vi "Buffer ArrayShellTest.vi"() -> ()   [LabVIEW 2014]
uses:
  <vilib>/measure/mamon.llb/Trigger Detection for 1 Channel.vi
  <vilib>/measure/NI_MAPro.lvlib
panel:
  out "Array":dbl[](array[numeric])
  out "trigger location":dbl
  out "index of element":i32
  out "Output Graph":dynamicdata(graph) caption="Sine"
  in  "stop":bool
  out "Output Array":dbl[](array[numeric])
  in  "Total amount of Pts":i32
  in  "Trigger Threshold":dbl
  out "SineGenerator":dynamicdata(graph) caption="Sine"
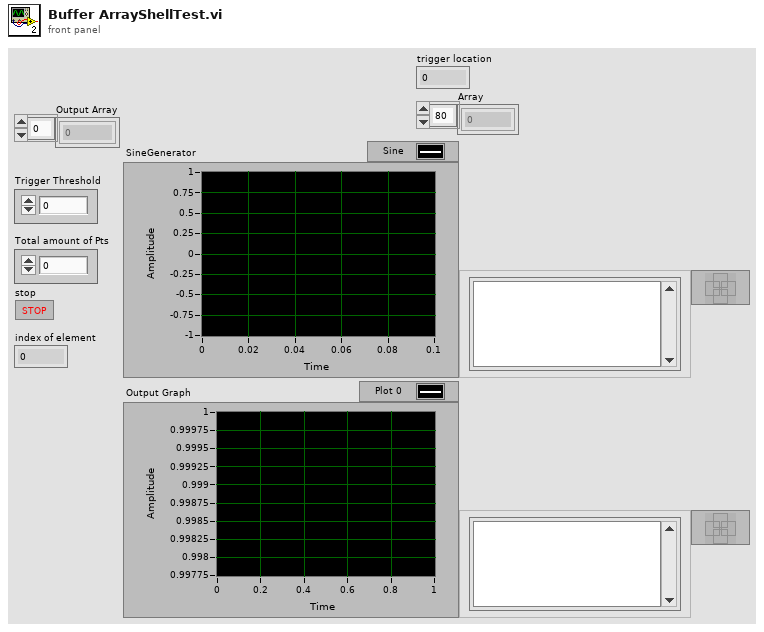
[diagram p1: front panel]
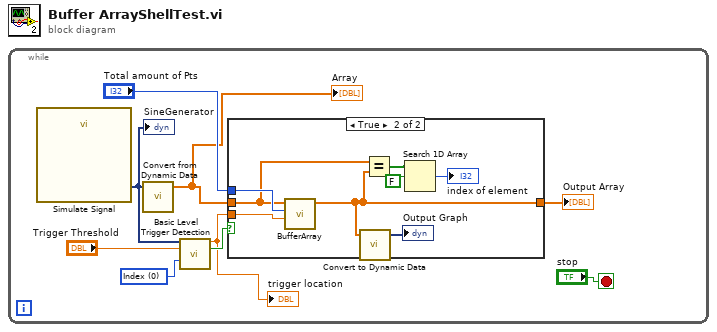
[diagram p0: block diagram]
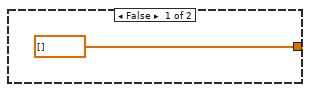
[diagram p2: hidden frame]
diagram:
  n1 = while {
    stop <- "stop" stop-if-true
    w6 = u16 0 items=["Index", "Time"] ("location mode")
    n2 = call "Simulate Signal"() -> ("Sine"=w8:dynamicdata)  [unwired: 14 in, 1 out]
    "SineGenerator" <- w8
    n3 = call "Convert from Dynamic Data"("Dynamic Data Type"=w8) -> ("Array"=w1:dbl[])  [unwired: 3 in]
    "Array" <- w1
    n4 = call-poly <vilib>:"Basic Level Trigger Detection.vi"("signal in"=w8, "level"="Trigger Threshold", "location mode"=w6) -> ("trigger location"=w2:dbl, "trigger detected?"=w5:bool)  [unwired: 10 in, 1 out]
    "trigger location" <- w2
    n5 = case shown="True" w5 {
      tunnel: "Total amount of Pts" -> [_ w18]
      tunnel: w2 -> [_ w17]
      tunnel: w1 -> [_ w11]
      tunnel: [dbl[] [] w15] -> w3
      frame False {
      }
      frame True {
        n6 = call "BufferArray.VI"("Index"=w17, "Total amount of Pts"=w18, "Input Y-values"=w11) -> ("Output Array"=w15:dbl[])  [unwired: 8 in]
        n7 = call "Convert to Dynamic Data"("Array"=w15) -> ("Dynamic Data Type"=→"Output Graph":dynamicdata)  [unwired: 3 in]
        n8 = Equal?(x=w11, y=w15) -> (x = y?=w14:bool[])
        n9 = Search 1D Array(1D array=w14, element=FALSE) -> (index of element=→"index of element":i32)  [unwired: 1 in]
      }
    }
    "Output Array" <- w3
  }
